vi "IV data file names.vi"(11 "book number":i32) -> (1 "x axis":string, 2 "Field":string, 3 "IV":string)   [LabVIEW 2024]
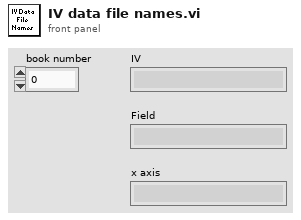
[diagram p1: front panel]
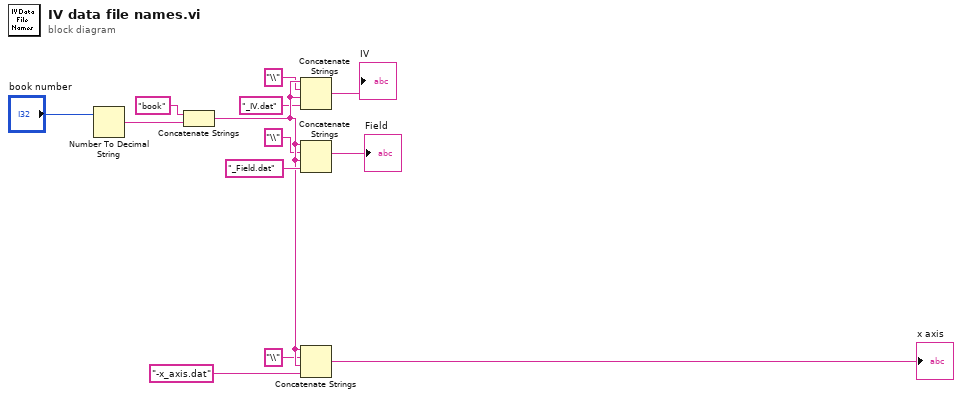
[diagram p0: block diagram]
diagram:
  n1 = Number To Decimal String(number="book number") -> (decimal integer string=w1:string)  [unwired: 1 in]
  n2 = Concatenate Strings("book" ("string"), w1) -> (w10:string)
  n3 = Concatenate Strings(w10, "\\" ("string"), w10, "_IV.dat" ("string")) -> (→"IV":string)
  n4 = Concatenate Strings(w10, "\\" ("string"), w10, "_Field.dat" ("string")) -> (→"Field":string)
  n5 = Concatenate Strings(w10, "\\" ("string"), w10, "-x_axis.dat" ("string")) -> (→"x axis":string)
